vi "sub1.vi"() -> ()   [LabVIEW 2020]
panel:
  out "Process Temps":dbl(graph)
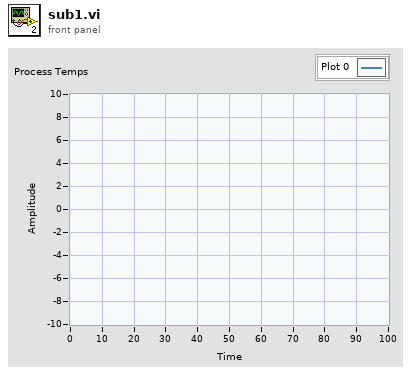
[diagram p1: front panel]
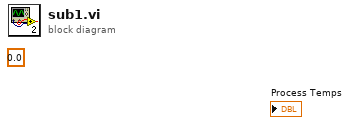
[diagram p0: block diagram]
diagram:
  (unwired) 0.0
